vi "simulateData(SubVI).vi"() -> (0 "output cluster":T1)   [LabVIEW 2010]
uses:
  CPES/types/OutputDataFormat.ctl
  CPES/types/VarableID.ctl
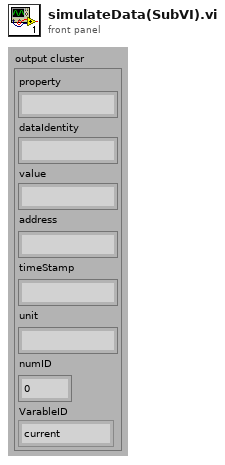
[diagram p1: front panel]
types:
  T1 = typedef "OutputDataFormat.ctl" = cluster{"property":string, "dataIdentity":string, "value":string, "address":string, "timeStamp":string, "unit":string, "numID":i32, "VarableID":T2}
  T2 = typedef "VarableID.ctl" = enum16{"current", "power", "PF", "voltage"}
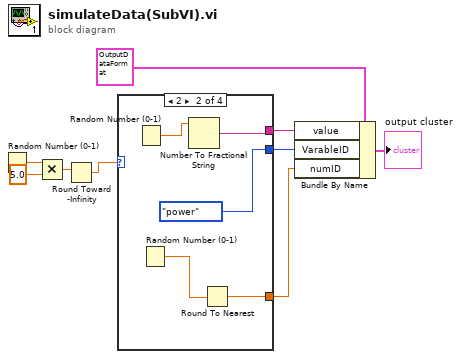
[diagram p0: block diagram]
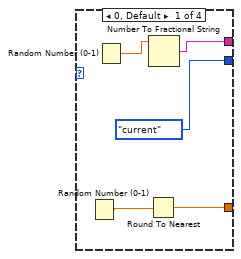
[diagram p2: hidden frame]
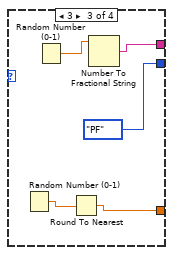
[diagram p3: hidden frame]
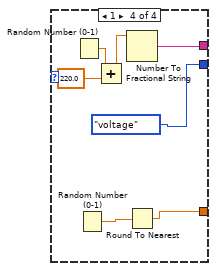
[diagram p4: hidden frame]
diagram:
  n1 = Random Number (0-1)() -> (number: 0 to 1=w5:dbl)
  n2 = Multiply(x=w5, y=5.0) -> (x*y=w7:dbl)
  n3 = Round Toward -Infinity(1:w7) -> (0:w8:dbl)
  n4 = case shown="2" w8 {
    tunnel: [w13 w19 w24 w31] -> w3
    tunnel: [VarableID."current" ("VarableID") VarableID."power" ("VarableID") VarableID."PF" ("VarableID") VarableID."voltage" ("VarableID")] -> w4
    tunnel: [w12 w17 w22 w29] -> w9
    frame 0, Default {
      n5 = Random Number (0-1)() -> (number: 0 to 1=w10:dbl)
      n6 = Random Number (0-1)() -> (number: 0 to 1=w11:dbl)
      n7 = Round To Nearest(number=w10) -> (nearest integer value=w12:dbl)
      n8 = Number To Fractional String(number=w11) -> (F-format string=w13:string)  [unwired: 3 in]
    }
    frame 2 {
      n9 = Random Number (0-1)() -> (number: 0 to 1=w16:dbl)
      n10 = Random Number (0-1)() -> (number: 0 to 1=w15:dbl)
      n11 = Number To Fractional String(number=w16) -> (F-format string=w19:string)  [unwired: 3 in]
      n12 = Round To Nearest(number=w15) -> (nearest integer value=w17:dbl)
    }
    frame 3 {
      n13 = Random Number (0-1)() -> (number: 0 to 1=w20:dbl)
      n14 = Random Number (0-1)() -> (number: 0 to 1=w21:dbl)
      n15 = Round To Nearest(number=w20) -> (nearest integer value=w22:dbl)
      n16 = Number To Fractional String(number=w21) -> (F-format string=w24:string)  [unwired: 3 in]
    }
    frame 1 {
      n17 = Random Number (0-1)() -> (number: 0 to 1=w27:dbl)
      n18 = Random Number (0-1)() -> (number: 0 to 1=w28:dbl)
      n19 = Add(x=w27, y=220.0) -> (x+y=w25:dbl)
      n20 = Number To Fractional String(number=w25) -> (F-format string=w31:string)  [unwired: 3 in]
      n21 = Round To Nearest(number=w28) -> (nearest integer value=w29:dbl)
    }
  }
  n22 = Bundle By Name(cluster=T1 {"property"="", "dataIdentity"="电流", "value"="10", "address"="01000000", "timeStamp"="", "unit"="A", "numID"=1, "VarableID"=enum."current"} ("CommandText"), "value"=w3, "VarableID"=w4, "numID"=w9) -> (→"output cluster":T1)
